vi "test_theory_data_vis.vi"() -> ()   [LabVIEW 2021]
panel:
  out "Waveform Graph 2":dbl[](graph)
  in  "stop":bool
  out "Waveform Graph":dbl[](graph)
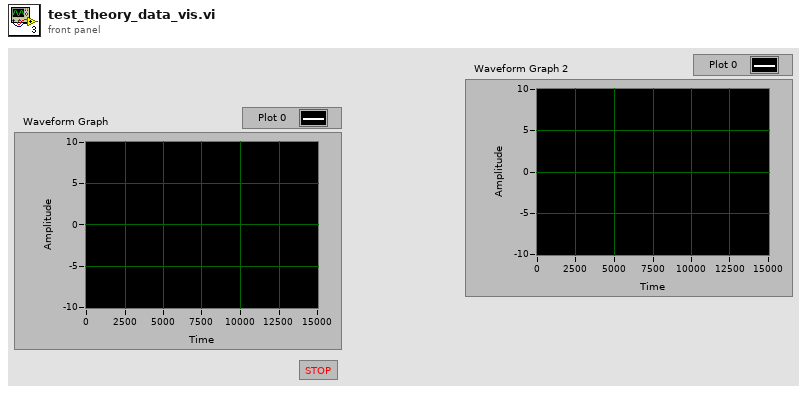
[diagram p1: front panel]
types:
  T1 = cluster{"Accelorometer":dbl[], "Displacement":dbl[], "dt":dbl, "Final Time":dbl}
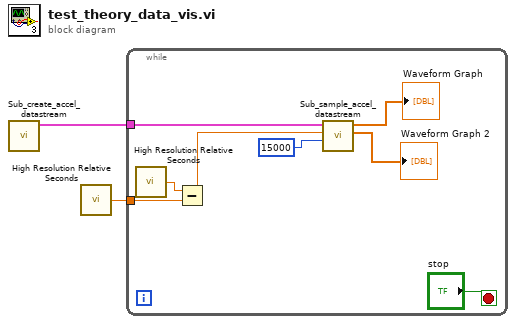
[diagram p0: block diagram]
diagram:
  n1 = call "Sub_create_accel_datastream.vi"() -> ("Experimental Replay"=w1:T1)  [unwired: 9 in, 2 out]
  n2 = call <vilib>:"High Resolution Relative Seconds.vi"() -> ("relative seconds"=w2:dbl)
  n3 = while {
    tunnel: w2 -> [w6]
    tunnel: w1 -> [w4]
    stop <- "stop" stop-if-true
    n4 = call <vilib>:"High Resolution Relative Seconds.vi"() -> ("relative seconds"=w5:dbl)
    n5 = Subtract(x=w5, y=w6) -> (x-y=w7:dbl)
    n6 = call "Sub_sample_accel_datastream.vi"("FFT data length"=15000, "Simulation Time"=w7, "Experimental Replay"=w4) -> ("Displacment sample"=→"Waveform Graph 2":dbl[], "Accelerometer sample"=→"Waveform Graph":dbl[])  [unwired: 7 in]
  }
